vi "LoadApp.vi"(3 "error in (no error)":errorcluster, 4 "Demo?":bool, 5 "Status Notifier":refnum<notifier>) -> (0 "error out":errorcluster)   [LabVIEW 2020]
uses:
  ViewController/Microscope Controller/MicroscopeController.lvclass
  C:/Program Files/National Instruments/LabVIEW 2020/vi.lib/ActorFramework/Actor/Actor.lvclass
  <vilib>/ActorFramework/Actor/Actor.lvclass
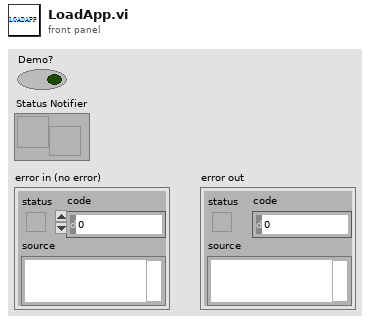
[diagram p1: front panel]
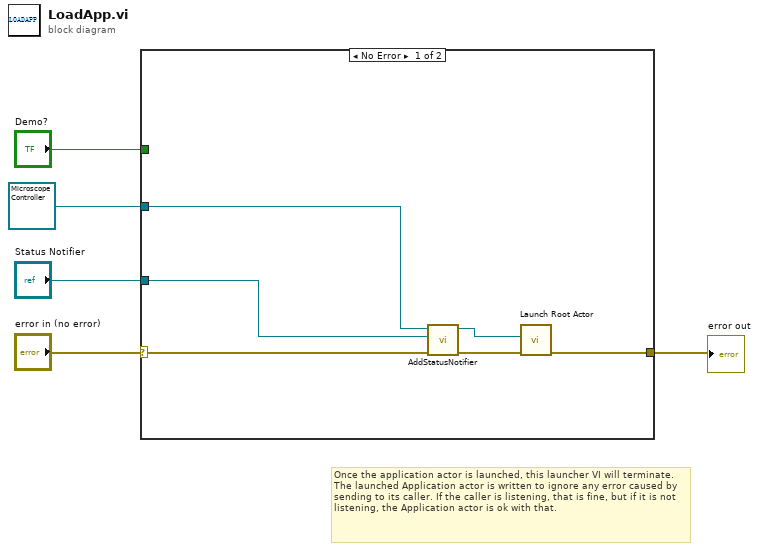
[diagram p0: block diagram]
diagram:
  # "Once the application actor is launched, this launcher VI will terminate. The launched Application actor is written to ignore any error caused by sending to its caller. If the caller is listening, that is fine, but if it is not listening, the Application actor is ok with that."
  n1 = case shown="No Error" "error in (no error)" {
    selector: "error in (no error)" -> [w11 w12]
    tunnel: "Demo?" -> [_ _]
    tunnel: refnum<class "MicroscopeController.lvclass"> refnum ("MicroscopeController.lvlib:MicroscopeController.lvclass") -> [w6 _]
    tunnel: [w10 w12] -> w3
    tunnel: "Status Notifier" -> [w7 _]
    frame No Error {
      n2 = call-dynamic "AddStatusNotifier.vi"("error in (no error)"=w11, "Status Notifier"=w7, "MicroscopeController in"=w6) -> ("error out"=w9:errorcluster, "MicroscopeController out"=w8:refnum<class "MicroscopeController.lvclass">)  [unwired: 7 in]
      n3 = call <vilib>:"Launch Root Actor.vi"("error in (no error)"=w9, "Actor"=w8) -> ("error out"=w10:errorcluster)  [unwired: 8 in, 1 out]
    }
    frame Error {
    }
  }
  "error out" <- w3
